vi "Method.vi"(4 "Value B":refnum<class "Abs_Numeric.lvclass">, 5 "Value A":refnum<class "Abs_Complex Double Float.lvclass">) -> (1 "Result":refnum<class "Abs_Boolean.lvclass">)   [LabVIEW 2021, in "Not Equal_CPLX_DBL.lvclass"]
uses:
  Not Equal_CPLX_DBL.lvclass
  Abs_Types/Complex Double Float/Abs_Complex Double Float.lvclass
  Abs_Types/Boolean/Abs_Boolean.lvclass
  Abs_Types/Numeric/Abs_Numeric.lvclass
  C:/TSA/LV_Abstract/Source/Functions/Support/Compare/Two Term/CPLX_DBL/AbsComp_Two Term_CPLX_DBL.lvclass
  C:/Program Files (x86)/National Instruments/LabVIEW 2021/vi.lib/TSA/Abstract Data Classes/Abs_Types/Boolean/Abs_Boolean.lvclass
  Support/Compare/Two Term/CPLX_DBL/AbsComp_Two Term_CPLX_DBL.lvclass/AbsComp_Two Term_CPLX_DBL.ctl
  Support/Compare/Two Term/CPLX_DBL/Properties/Write Numeric A.vi
  Support/Compare/Two Term/CPLX_DBL/Properties/Write Numeric B.vi
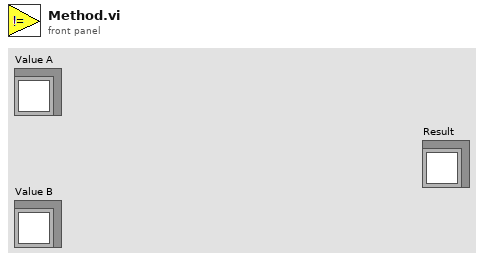
[diagram p1: front panel]
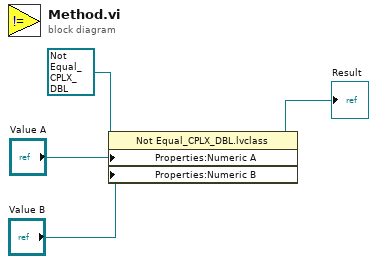
[diagram p0: block diagram]
diagram:
  n1 = property class="Not Equal_CPLX_DBL.lvclass"(reference=refnum<class "Not Equal_CPLX_DBL.lvclass"> refnum ("Greater 0_U64.lvclass"), "Properties:Numeric A"="Value A", "Properties:Numeric B"="Value B") -> (reference out=→"Result":refnum<class "Not Equal_CPLX_DBL.lvclass">)  [unwired: 1 in, 1 out]
